vi "张嘉欣.vi"(1 "b":dbl, 2 "a":dbl) -> (0 "波形图":dbl[][](graph))   [LabVIEW 2017]
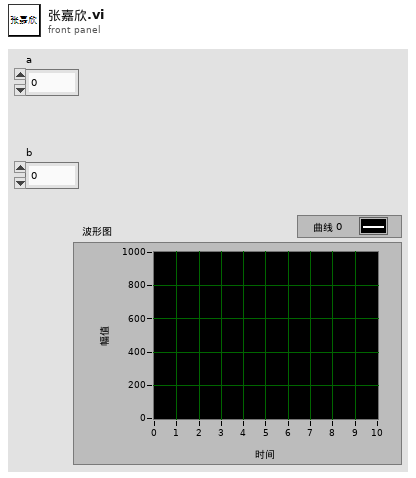
[diagram p1: front panel]
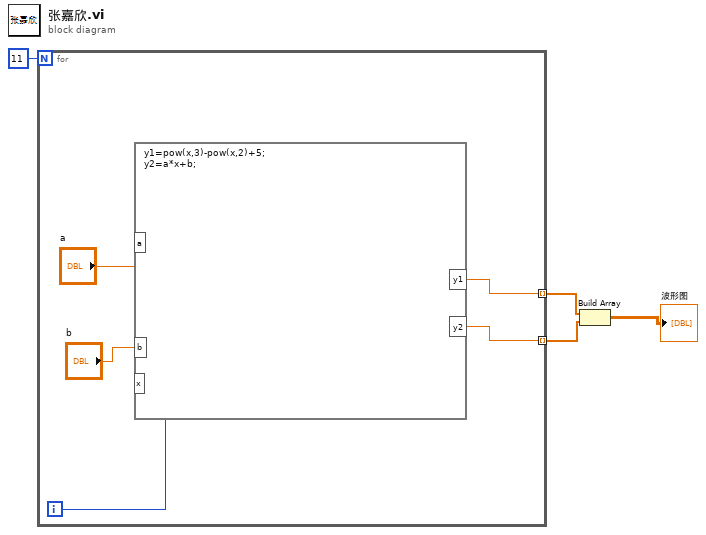
[diagram p0: block diagram]
diagram:
  n1 = for {
    N: 11 -> [_]
    tunnel: [w7] -> w3 mode=indexing
    tunnel: [w6] -> w2 mode=indexing
    i -> [w5]
    n2 = formula code="y1=pow(x,3)-pow(x,2)+5;\ny2=a*x+b;"("a"="a", "b"="b", "x"=w5) -> ("y1"=w7:dbl, "y2"=w6:dbl)
  }
  n3 = Build Array(w3, w2) -> (→"波形图":dbl[][])
